vi "Walsh Hadamard PtByPt (obs 85).vi"(2 "initialize":bool, 3 "sample length":i32=128, 5 "x":dbl format="%0.2f") -> (0 "error":i32, 1 "Walsh Hadamard {X}":dbl[](array[numeric]))   [LabVIEW 2020, in "NI_PtbyPt.lvlib"]
doc: "Performs the real Walsh Hadamard transform."
uses:
  NI_PtbyPt.lvlib
  NI_Gmath.lvlib
panel:
  # "This VI is obsolete !!!\nYou should replace this VI in your diagram with the Walsh \nHadamard PtByPt VI.\n\nNOTE: Please be aware of that the new Walsh Hadamard\n           PtByPt VI is set to reentrant."
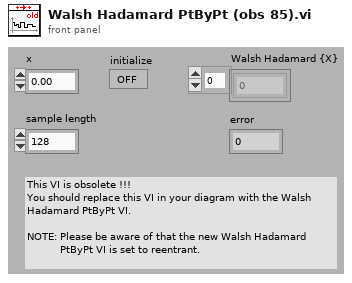
[diagram p1: front panel]
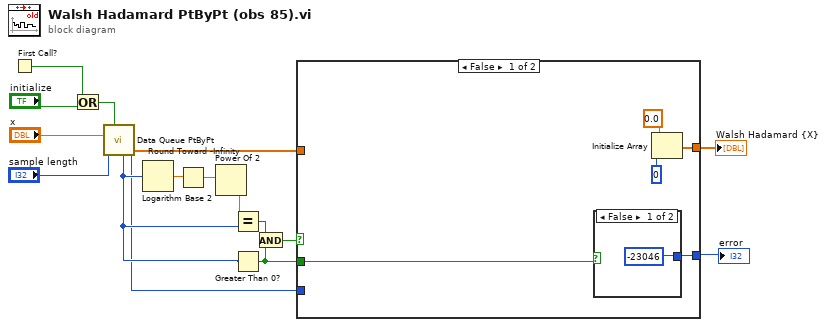
[diagram p0: block diagram]
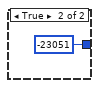
[diagram p2: hidden frame]
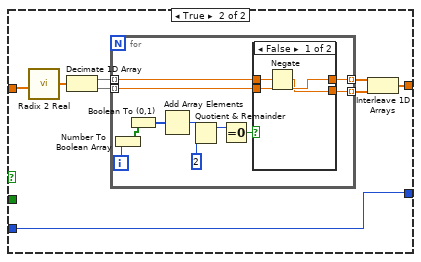
[diagram p3: hidden frame]
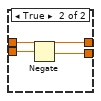
[diagram p4: hidden frame]
diagram:
  n1 = First Call?() -> (First Call?: T/F=w1:bool)
  n2 = Or(x=w1, y="initialize") -> (x .or. y?=w3:bool)
  n3 = call "Data Queue PtByPt.vi"("initialize"=w3, "sample length"="sample length", "input data point"="x") -> ("error"=w4:i32, "Current Queue"=w6:dbl[], "current length"=w5:i32)  [unwired: 4 in, 2 out]
  n4 = Logarithm Base 2(1:w5) -> (0:w14:dbl)
  n5 = Round Toward -Infinity(1:w14) -> (0:w13:dbl)
  n6 = Power Of 2(x=w13) -> (2^x=w12:dbl)
  n7 = Equal?(x=w12, y=w5) -> (x = y?=w11:bool)
  n8 = Greater Than 0?(x=w5) -> (x > 0?=w9:bool)
  n9 = And(x=w11, y=w9) -> (x .and. y?=w10:bool)
  n10 = case shown="False" w10 {
    tunnel: w6 -> [_ w31]
    tunnel: [w19 w25] -> w16
    tunnel: [w18 w24] -> w15
    tunnel: w9 -> [w17 _]
    tunnel: w4 -> [_ w24]
    frame False {
      n11 = case shown="False" w17 {
        tunnel: [-23046 -23051] -> w18
        frame False {
        }
        frame True {
        }
      }
      n12 = Initialize Array(0.0, 0) -> (w19:dbl[])
    }
    frame True {
      n13 = call "Radix 2 Real.vi"("X"=w31) -> ("Y"=w26:dbl[])
      n14 = Decimate 1D Array(w26) -> (w27:dbl[], w28:dbl[])
      n15 = for {
        tunnel: w27 -> [w35] mode=indexing
        tunnel: w28 -> [w34] mode=indexing
        tunnel: [w33] -> w29 mode=indexing
        tunnel: [w32] -> w30 mode=indexing
        i -> [w42]
        n16 = Number To Boolean Array(number=w42) -> (Boolean array=w41:bool[])
        n17 = Boolean To (0,1)(Boolean=w41) -> (0, 1=w40:i16[])
        n18 = Add Array Elements(numeric array=w40) -> (sum=w38:i16)
        n19 = Quotient & Remainder(x=w38, y=2) -> (x-y*floor(x/y)=w37:i32)  [unwired: 1 out]
        n20 = Equal To 0?(x=w37) -> (x = 0?=w36:bool)
        n21 = case shown="False" w36 {
          tunnel: w35 -> [w45 w48]
          tunnel: w34 -> [w44 w47]
          tunnel: [w44 w48] -> w33
          tunnel: [w43 w46] -> w32
          frame False {
            n22 = Negate(x=w45) -> (-x=w43:dbl)
          }
          frame True {
            n23 = Negate(x=w47) -> (-x=w46:dbl)
          }
        }
      }
      n24 = Interleave 1D Arrays(w29, w30) -> (w25:dbl[])
    }
  }
  "Walsh Hadamard {X}" <- w16
  "error" <- w15
